vi "Open_VI_and_Library_References.vi"(8 "error in (no error)":errorcluster, 11 "Build in":refnum<class "AB_Build.lvclass">) -> (0 "error out":errorcluster, 1 "VI refnums":refnum<vi>[](array[refnum]), 2 "library refnums":refnum<vi>[](array[refnum]), 3 "Build out":refnum<class "AB_Build.lvclass">, 4 "indexVIs":i32[](array[numeric]), 5 "indexLibraries":i32[](array[numeric]))   [LabVIEW 2020, in "AB_Build.lvclass"]
uses:
  <vilib>/AppBuilder/AB_Classes/Build/AB_Build.lvclass
  <vilib>/AppBuilder/AB_Classes/Build/AB_Build.lvclass/AB_Build.ctl
  <vilib>/AppBuilder/AB_Classes/Source/AB_Source.lvclass
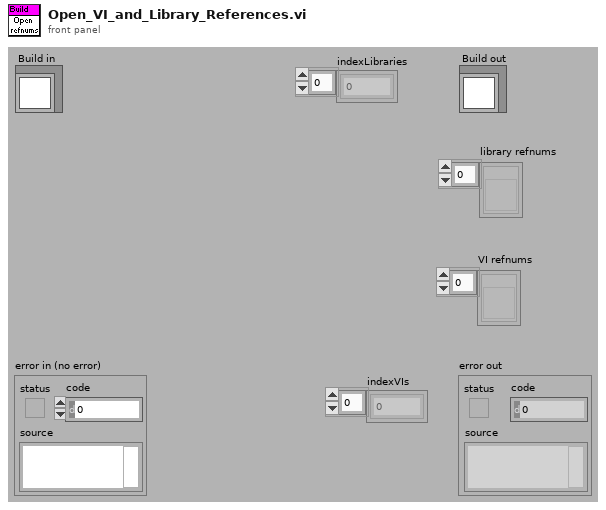
[diagram p1: front panel]
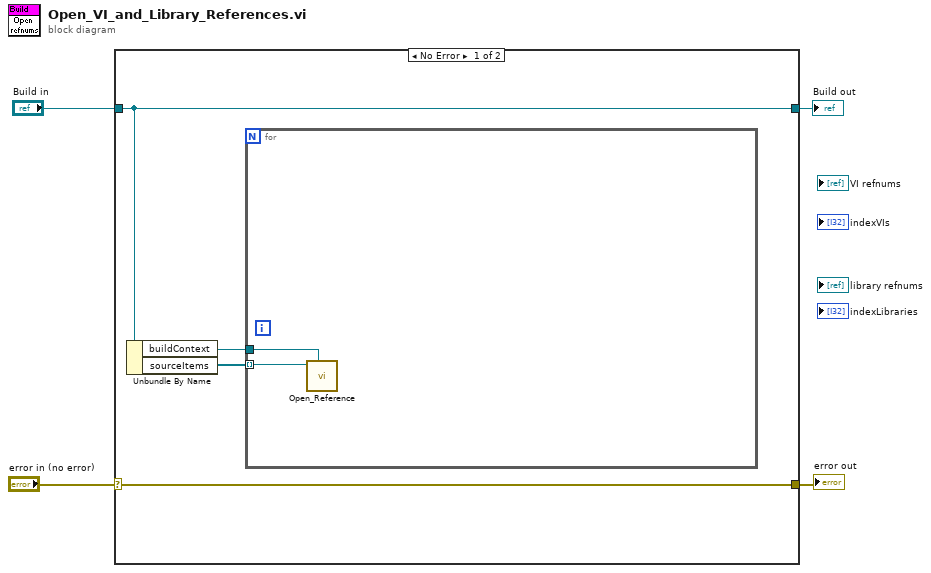
[diagram p0: block diagram]
diagram:
  n1 = case shown="No Error" "error in (no error)" {
    selector: "error in (no error)" -> [w8 w12]
    tunnel: [w8 w12] -> w3
    tunnel: [w7 w11] -> w1
    tunnel: "Build in" -> [w7 w11]
    frame No Error {
      n2 = Unbundle By Name(w7) -> ("buildContext"=w5:refnum<vi>, "sourceItems"=w6:refnum<class "AB_Source.lvclass">[])
      n3 = for {
        tunnel: w6 -> [w10] mode=indexing
        tunnel: w5 -> [w9]
        n4 = call-dynamic "Open_Reference.vi"("buildContext"=w9, "AB_Source in"=w10) -> ()  [unwired: 8 in, 2 out]
      }
    }
    frame Error {
    }
  }
  "error out" <- w3
  "Build out" <- w1
